vi "Convert Joystick Hat Event Data.vi"(11 "Event Data":u8[](array[numeric]) format="%.0x") -> (3 "Joystick Hat Event":T1 {"Which" format="%.0x"; "Type" format="%.0x"})   [LabVIEW 2019, in "LibSDL2.lvlib"]
uses:
  LibSDL2.lvlib
  Controls/Joysitck Hat Event.ctl
  Controls/Joystick Hat Value.ctl
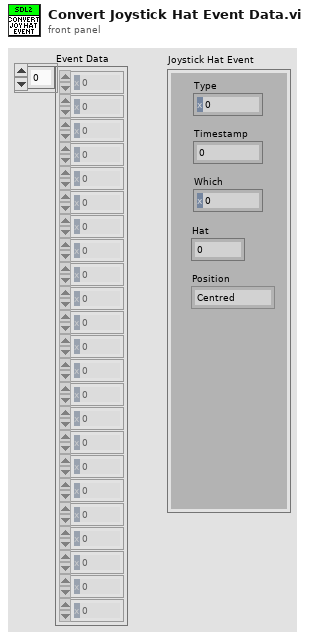
[diagram p1: front panel]
types:
  T1 = typedef "LibSDL2.lvlib/Joysitck Hat Event.ctl" = cluster{"Type":u32, "Timestamp":u32, "Which":i32, "Hat":u8, "Position":T2}
  T2 = typedef "LibSDL2.lvlib/Joystick Hat Value.ctl" = enum16{"Centred", "Up", "Right", "Down", "Left", "Right Up", "Right Down", "Left Up", "Left Down"}
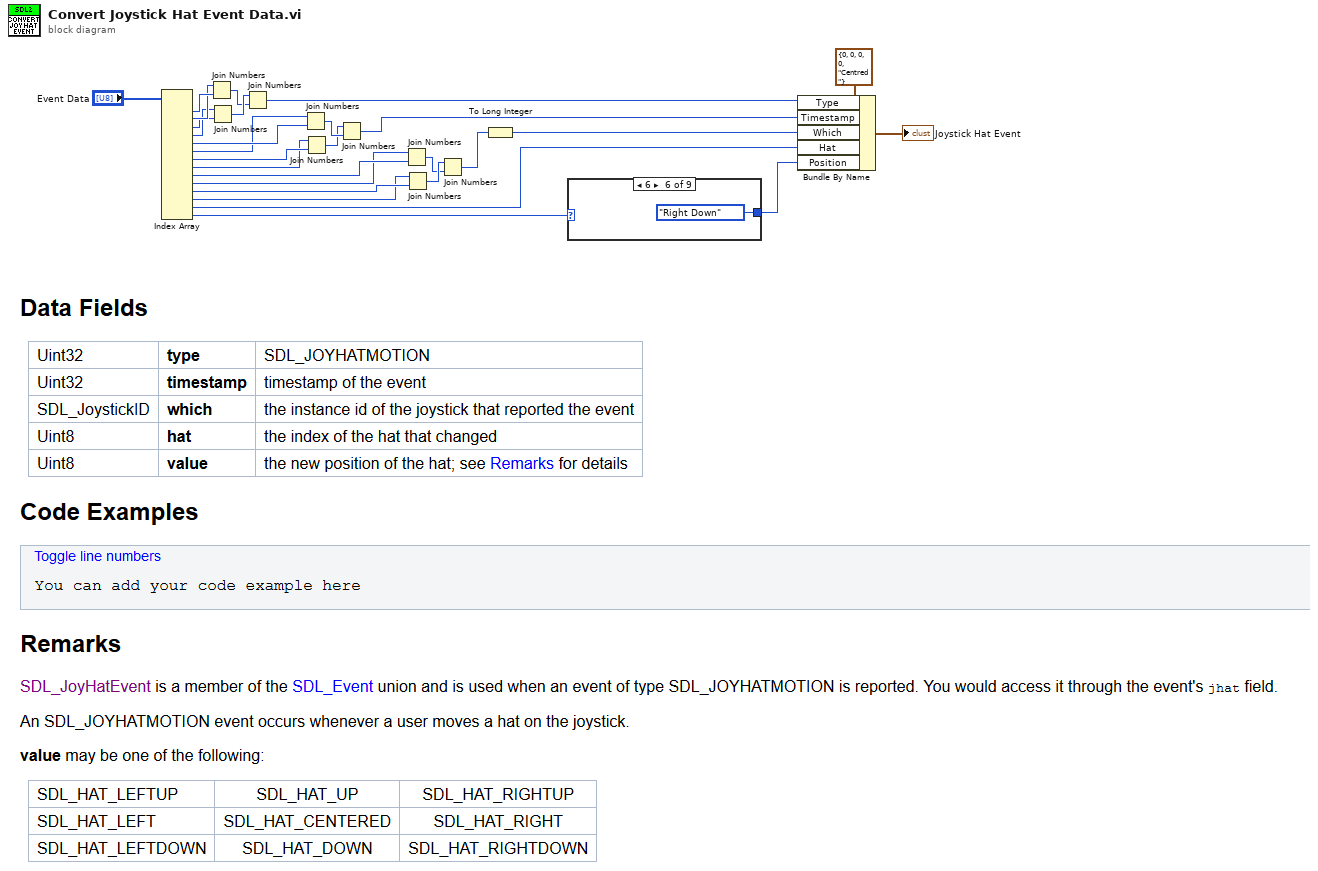
[diagram p0: block diagram]
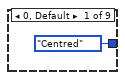
[diagram p2: hidden frame]
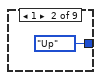
[diagram p3: hidden frame]
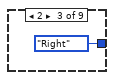
[diagram p4: hidden frame]
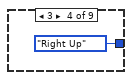
[diagram p5: hidden frame]
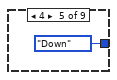
[diagram p6: hidden frame]
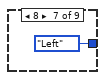
[diagram p7: hidden frame]
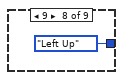
[diagram p8: hidden frame]
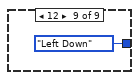
[diagram p9: hidden frame]
diagram:
  n1 = Index Array(array="Event Data") -> (element #1=w26:u8, element #2=w25:u8, element #3=w23:u8, element #4=w24:u8, element #5=w17:u8, element #6=w16:u8, element #7=w15:u8, element #8=w14:u8, element #9=w10:u8, element #10=w9:u8, element #11=w8:u8, element #12=w7:u8, element #13=w6:u8, element #14=w2:u8)  [unwired: 14 in]
  n2 = Join Numbers(hi=w25, lo=w26) -> ((hi.lo)=w21:u16)
  n3 = Join Numbers(hi=w24, lo=w23) -> ((hi.lo)=w22:u16)
  n4 = Join Numbers(hi=w22, lo=w21) -> ((hi.lo)=w20:u32)
  n5 = Join Numbers(hi=w16, lo=w17) -> ((hi.lo)=w19:u16)
  n6 = Join Numbers(hi=w14, lo=w15) -> ((hi.lo)=w18:u16)
  n7 = Join Numbers(hi=w18, lo=w19) -> ((hi.lo)=w13:u32)
  n8 = Join Numbers(hi=w9, lo=w10) -> ((hi.lo)=w11:u16)
  n9 = Join Numbers(hi=w7, lo=w8) -> ((hi.lo)=w12:u16)
  n10 = Join Numbers(hi=w12, lo=w11) -> ((hi.lo)=w5:u32)
  n11 = To Long Integer(number=w5) -> (32bit integer=w4:i32)
  n12 = case shown="6" w2 {
    tunnel: [Joystick_Hat_Value."Centred" ("Position") Joystick_Hat_Value."Up" ("Position") Joystick_Hat_Value."Right" ("Position") Joystick_Hat_Value."Right Up" ("Position") Joystick_Hat_Value."Down" ("Position") Joystick_Hat_Value."Right Down" ("Position") Joystick_Hat_Value."Left" ("Position") Joystick_Hat_Value."Left Up" ("Position") Joystick_Hat_Value."Left Down" ("Position")] -> w1
    frame 0, Default {
    }
    frame 1 {
    }
    frame 2 {
    }
    frame 3 {
    }
    frame 4 {
    }
    frame 6 {
    }
    frame 8 {
    }
    frame 9 {
    }
    frame 12 {
    }
  }
  n13 = Bundle By Name(cluster=T1 {"Type"=0, "Timestamp"=0, "Which"=0, "Hat"=0, "Position"=enum."Centred"} ("Joystick Hat Event"), "Type"=w20, "Timestamp"=w13, "Which"=w4, "Hat"=w6, "Position"=w1) -> (→"Joystick Hat Event":T1)
